vi "WAM_UserInput_Popup.vi"(0 "Enable":bool=TRUE, 5 "error in (no error)":errorcluster, 11 "UseBcScanner(t)":bool=TRUE) -> (8 "EmpName":string caption="Revision", 10 "UserString":string="062218\r\n", 12 "operator infor header":string, 14 "UserInput_Popup_refOut":refnum<vi>, 17 "UserBCPopup_ref_out":refnum<vi>, 18 "OK":bool, 19 "error out":errorcluster)   [LabVIEW 2018]
doc: "Displays a standard dialog box that prompts users to enter information, such as a user name and password.\n--------------------\n\nThis Express VI is configured as follows:\n\nMessage to Display to the User:"
panel:
  out "index of element":i32=-1
  in  "EmpLocation":string(combo) caption="LotID"
  in  "EmpName":string caption="Revision"
  in  "EmpID#":string caption="PN"
  out "String":string
  in  "Cancel":bool=TRUE
  in  "OK2":bool
  in  "OK1":bool=TRUE
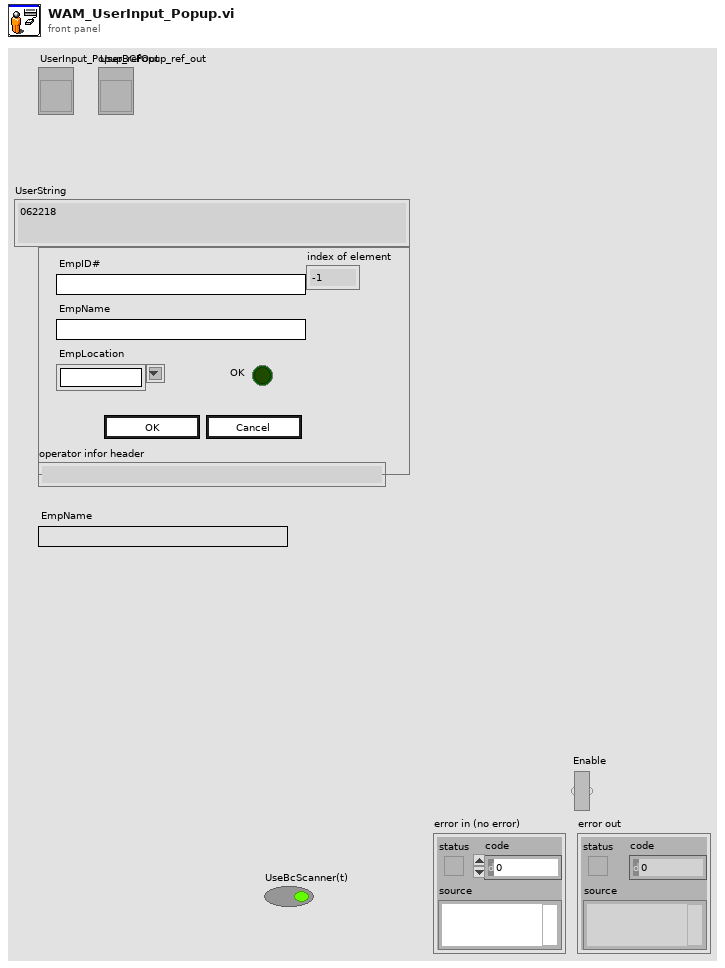
[diagram p1: front panel]
types:
  T1 = cluster{"Input Name":string, "Input Data Type":i32}[]
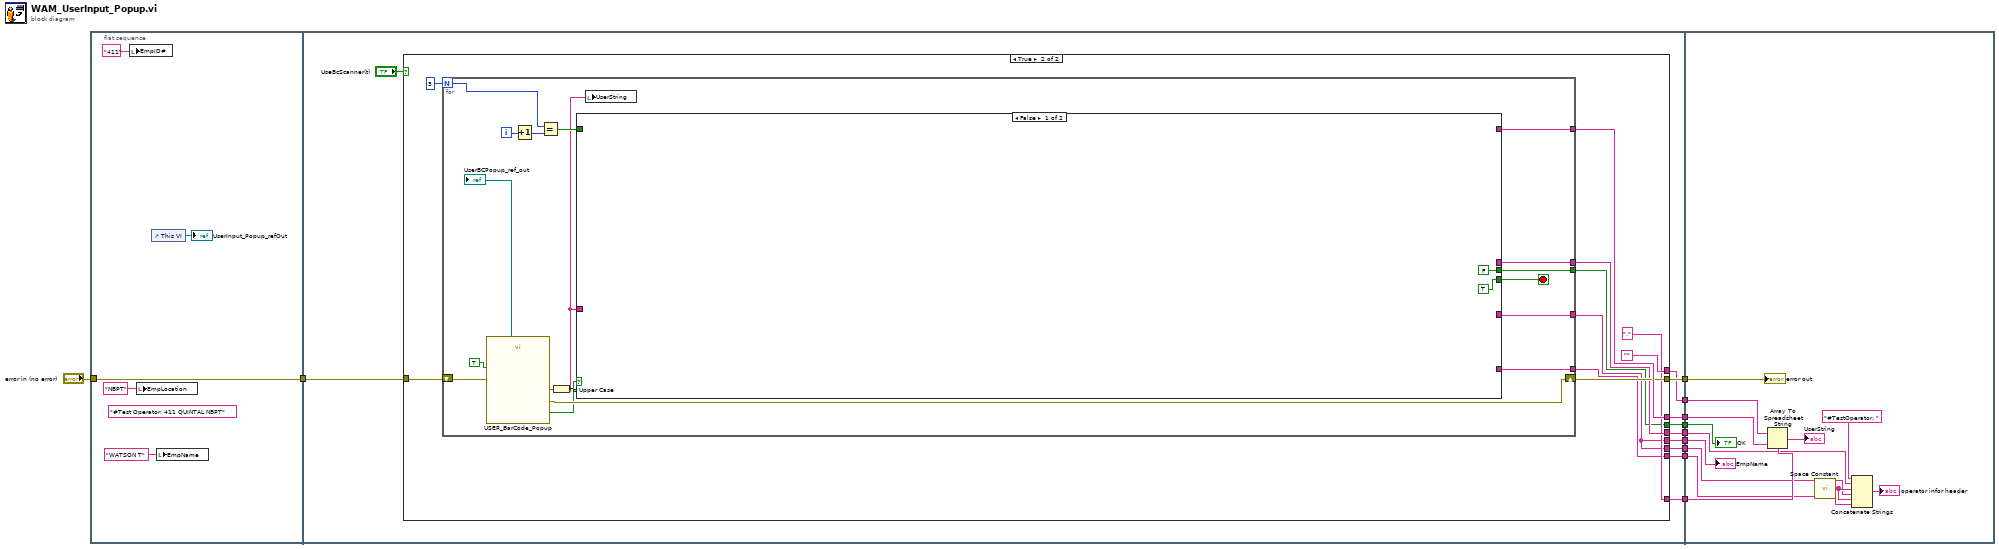
[diagram p0: block diagram]
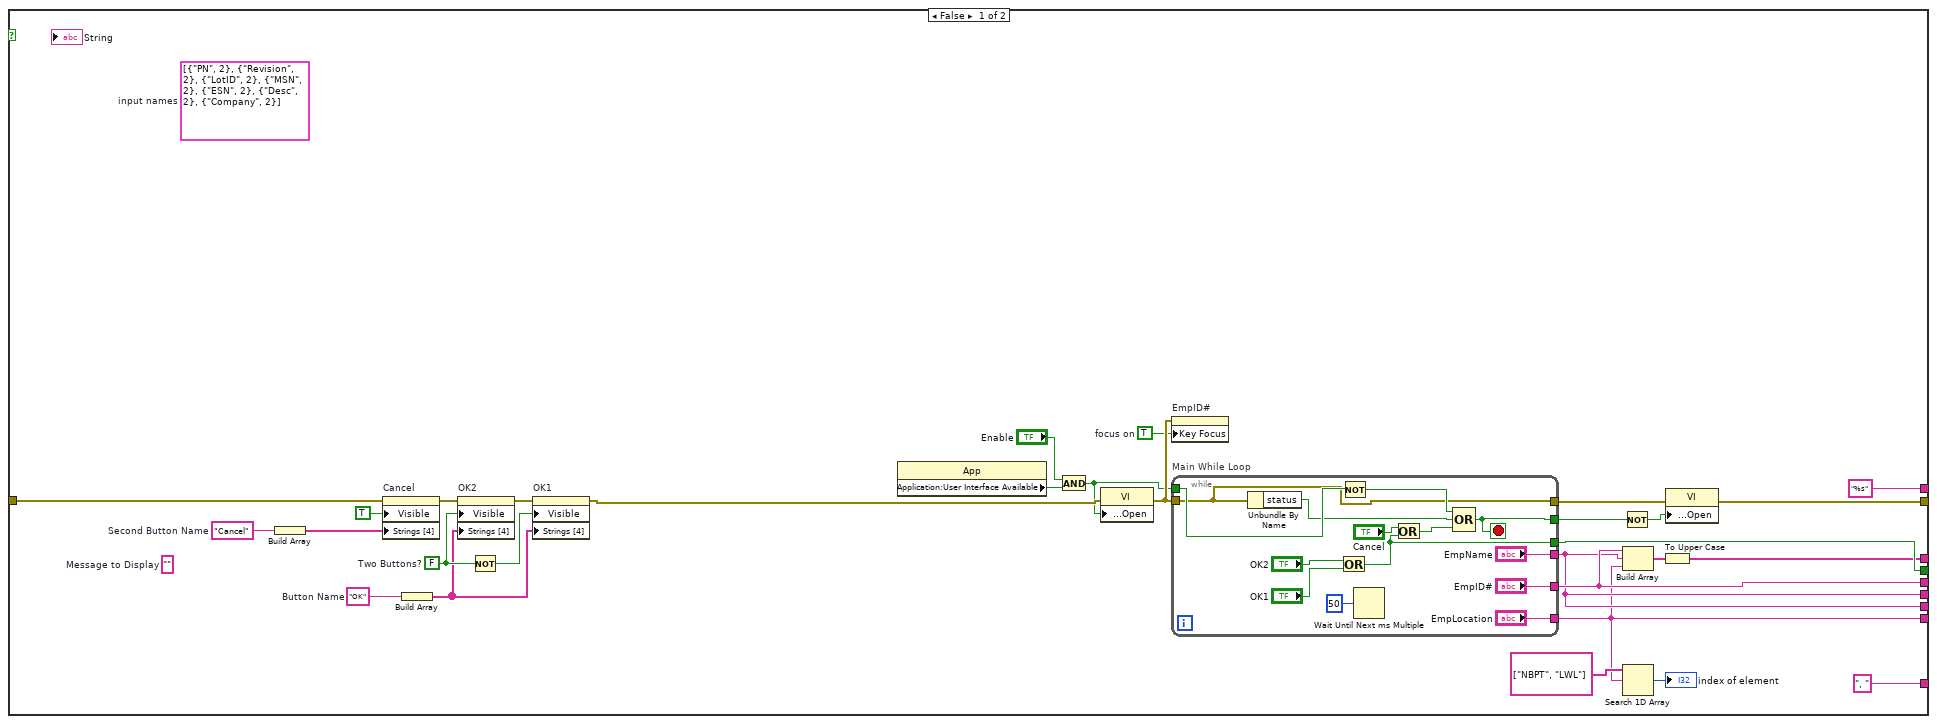
[diagram p2: hidden frame]
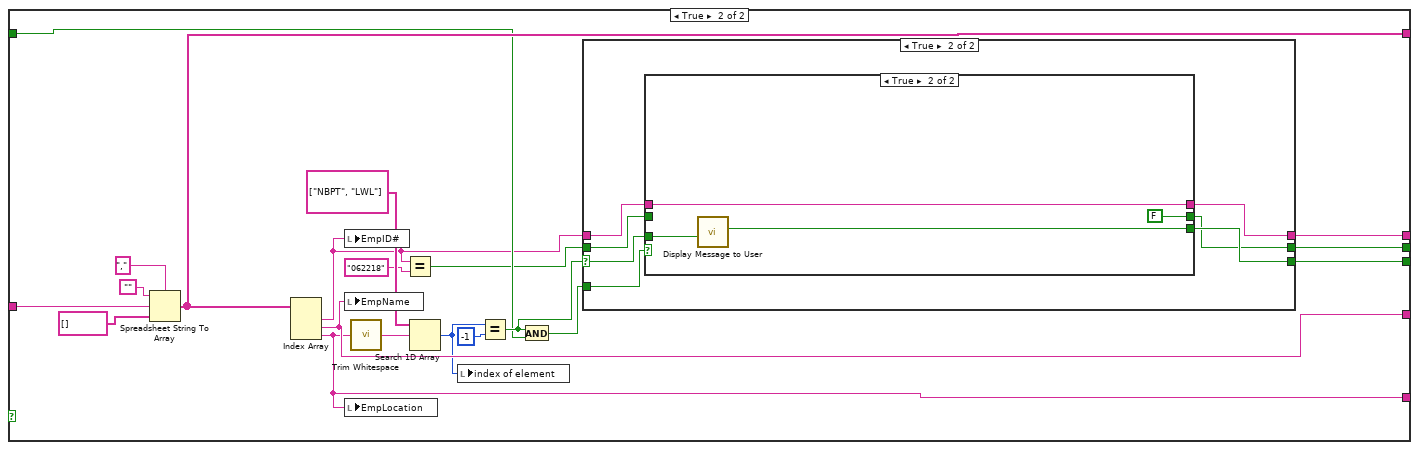
[diagram p3: hidden frame]
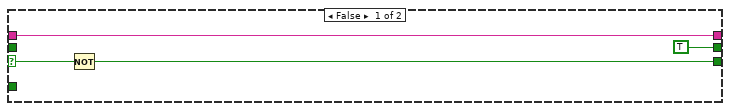
[diagram p4: hidden frame]
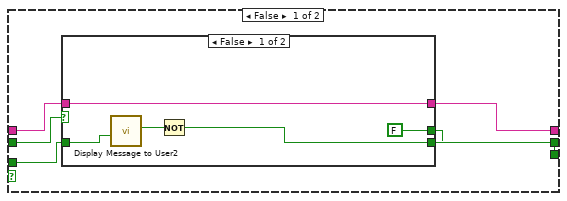
[diagram p5: hidden frame]
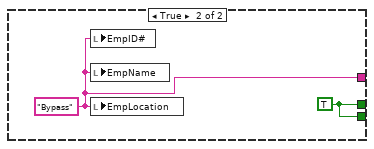
[diagram p6: hidden frame]
diagram:
  n1 = flat-sequence {
    tunnel: "error in (no error)" -> [w16]
    tunnel: [w16] -> w10
    tunnel: w10 -> [w27]
    tunnel: [w26] -> w9
    tunnel: [w25] -> w8
    tunnel: [w24] -> w7
    tunnel: [w23] -> w6
    tunnel: [w22] -> w5
    tunnel: [w20] -> w4
    tunnel: [w19] -> w3
    tunnel: [w18] -> w2
    tunnel: [w17] -> w1
    tunnel: w9 -> [w160]
    tunnel: w8 -> [w158]
    tunnel: w7 -> [w154]
    tunnel: w6 -> [w152]
    tunnel: w5 -> [w151]
    tunnel: w4 -> [w157]
    tunnel: w3 -> [w159]
    tunnel: w2 -> [w156]
    tunnel: w1 -> [w161]
    frame #0 {
      (unwired) "#Test Operator: 411 QUINTAL NBPT" ("OperatorInfo")
      n2 = local write "EmpID#"("411" ("PN")) -> ()
      n3 = local write "EmpLocation"("NBPT" ("LotID")) -> ()
      n4 = control-ref of="This VI"() -> (→"UserInput_Popup_refOut":refnum<vi>)
      n5 = local write "EmpName"("WATSON T" ("Revision")) -> ()
    }
    frame #1 {
      n6 = case shown="True" "UseBcScanner(t)" {
        tunnel: w27 -> [w45 w80]
        tunnel: [w43 w79] -> w26
        tunnel: [w28 w81] -> w25
        tunnel: [w36 w78] -> w24
        tunnel: [w33 w75] -> w23
        tunnel: [w31 w74] -> w22
        tunnel: ["%s" ("format string") "" ("format string")] -> w20
        tunnel: [", " ("delimiter (Tab)") "," ("delimiter (Tab)")] -> w19
        tunnel: [w33 w75] -> w18
        tunnel: [w29 w72] -> w17
        frame False {
          w39 = TRUE  # focus on
          (unwired) T1 [{"Input Name"="PN", "Input Data Type"=2}, {"Input Name"="Revision", "Input Data Type"=2}, {"Input Name"="LotID", "Input Data Type"=2}, {"Input Name"="MSN", "Input Data Type"=2}, {"Input Name"="ESN", "Input Data Type"=2}, {"Input Name"="Desc", "Input Data Type"=2}, {"Input Name"="Company", "Input Data Type"=2}]  # input names
          w50 = "Cancel"  # Second Button Name
          w48 = "OK"  # Button Name
          (unwired) ""  # Message to Display
          w57 = FALSE  # Two Buttons?
          n7 = Build Array(w50) -> (w51:string[])
          n8 = property on="Cancel" class="Bool"(error in=w45, "Visible"=TRUE, "Strings [4]"=w51) -> (error out=w55:errorcluster)  [unwired: 1 in, 1 out]
          n9 = Build Array(w48) -> (w49:string[])
          n10 = property on="OK2" class="Bool"(error in=w55, "Visible"=w57, "Strings [4]"=w49) -> (error out=w54:errorcluster)  [unwired: 1 in, 1 out]
          n11 = Not(x=w57) -> (.not. x?=w56:bool)
          n12 = property on="OK1" class="Bool"(error in=w54, "Visible"=w56, "Strings [4]"=w49) -> (error out=w47:errorcluster)  [unwired: 1 in, 1 out]
          n13 = property class="App"() -> ("Application:User Interface Available"=w40:bool)  [unwired: 2 in, 2 out]
          n14 = And(x="Enable", y=w40) -> (x .and. y?=w41:bool)
          n15 = property class="VI"(error in=w47, "Front Panel Window:Open"=w41) -> (error out=w46:errorcluster)  [unwired: 1 in, 1 out]
          n16 = property on="EmpID#" class="Str"(error in=w46, "Key Focus"=w39) -> ()  [unwired: 1 in, 2 out]
          n17 = while "Main While Loop" {
            tunnel: [w68] -> w29
            tunnel: w41 -> [w66]
            tunnel: [w64] -> w52
            tunnel: w46 -> [w63]
            tunnel: [w63] -> w44
            tunnel: ["EmpID#"] -> w36
            tunnel: ["EmpName"] -> w33
            tunnel: ["EmpLocation"] -> w31
            stop <- w64 stop-if-true
            n18 = Unbundle By Name(w63) -> ("status"=w61:bool)
            n19 = Or(x="OK2", y="OK1") -> (x .or. y?=w68:bool)
            n20 = Not(x=w66) -> (.not. x?=w65:bool)
            n21 = Wait Until Next ms Multiple(millisecond multiple=u32 50) -> ()  [unwired: 1 out]
            n22 = Or(x="Cancel", y=w68) -> (x .or. y?=w62:bool)
            n23 = Compound Arithmetic op=OR(w65, w61, w62) -> (w64:bool)
          }
          n24 = Not(x=w52) -> (.not. x?=w53:bool)
          n25 = Build Array(w36, w33, w31) -> (w38:string[])
          n26 = Search 1D Array(1D array=string[] ["NBPT", "LWL"], element=w31) -> (index of element=→"index of element":i32)  [unwired: 1 in]
          n27 = To Upper Case(1:w38) -> (0:w28:string[])
          n28 = property class="VI"(error in=w44, "Front Panel Window:Open"=w53) -> (error out=w43:errorcluster)  [unwired: 1 in, 1 out]
        }
        frame True {
          n29 = for {
            N: 3 -> [w91]
            tunnel: [w97] -> w81
            tunnel: [w88] -> w78
            tunnel: [w94] -> w75
            tunnel: [w93] -> w74
            shift-right: [w95] -> w79
            shift-left: w80 -> [w96]
            tunnel: [w85] -> w72
            i -> [w90]
            stop <- w87 stop-if-true
            n30 = call "USER_BarCode_Popup.vi"("Enable"=TRUE, "error in (no error)"=w96) -> ("UserBCPopup_ref_out"=→"UserBCPopup_ref_out":refnum<vi>, "Bar Code"=w84:string, "OK"=w86:bool, "error out"=w95:errorcluster)  [unwired: 14 in]
            n31 = Increment(x=w90) -> (x+1=w89:i32)
            n32 = Equal?(x=w91, y=w89) -> (x = y?=w92:bool)
            n33 = To Upper Case(1:w84) -> (0:w82:string)
            n34 = case shown="False" w86 {
              tunnel: w82 -> [_ w119]
              tunnel: [_ w117] -> w97
              tunnel: [_ w115] -> w94
              tunnel: [_ w113] -> w93
              tunnel: w92 -> [_ w108]
              tunnel: [_ w104] -> w88
              tunnel: [TRUE ("OK") w102] -> w87
              tunnel: [FALSE ("OK") w101] -> w85
              frame False {
              }
              frame True {
                n35 = Spreadsheet String To Array(delimiter (Tab)=",", format string="", spreadsheet string=w119, array type (2D Dbl)=string[] []) -> (array=w117:string[])
                n36 = Index Array(array=w117) -> (element #1=w103:string, element #2=w115:string, element #3=w113:string)  [unwired: 3 in]
                n37 = local write "EmpID#"(w103) -> ()
                n38 = local write "EmpName"(w115) -> ()
                n39 = local write "EmpLocation"(w113) -> ()
                n40 = call <vilib>:"Trim Whitespace.vi"("string"=w113) -> ("trimmed string"=w110:string)  [unwired: 1 in]
                n41 = Equal?(x=w103, y="062218") -> (x = y?=w105:bool)
                n42 = Search 1D Array(1D array=string[] ["NBPT", "LWL"], element=w110) -> (index of element=w112:i32)  [unwired: 1 in]
                n43 = local write "index of element"(w112) -> ()
                n44 = Equal?(x=w112, y=-1) -> (x = y?=w109:bool)
                n45 = And(x=w109, y=w108) -> (x .and. y?=w107:bool)
                n46 = case shown="True" w109 {
                  selector: w109 -> [w124 w131]
                  tunnel: [w123 w130] -> w102
                  tunnel: w107 -> [_ w129]
                  tunnel: w105 -> [_ w128]
                  tunnel: [w122 w127] -> w104
                  tunnel: w103 -> [w122 w126]
                  tunnel: [TRUE w125] -> w101
                  frame False {
                    n47 = Not(x=w124) -> (.not. x?=w123:bool)
                  }
                  frame True {
                    n48 = case shown="True" w129 {
                      tunnel: w131 -> [w137 w148]
                      tunnel: [w136 w147] -> w130
                      tunnel: w128 -> [w135 _]
                      tunnel: [w134 w146] -> w127
                      tunnel: w126 -> [w133 w146]
                      tunnel: [w132 FALSE] -> w125
                      frame False {
                        n49 = case shown="False" w135 {
                          tunnel: w137 -> [w142 _]
                          tunnel: [w140 w143] -> w136
                          tunnel: [w139 w144] -> w134
                          tunnel: w133 -> [w139 _]
                          tunnel: [FALSE w143] -> w132
                          frame False {
                            n50 = call "Display Message to User2"("Enable"=w142) -> ("OK"=w141:bool)  [unwired: 9 in, 1 out]
                            n51 = Not(x=w141) -> (.not. x?=w140:bool)
                          }
                          frame True {
                            w144 = "Bypass" ("EmpName")
                            w143 = TRUE
                            n52 = local write "EmpID#"(w144) -> ()
                            n53 = local write "EmpName"(w144) -> ()
                            n54 = local write "EmpLocation"(w144) -> ()
                          }
                        }
                      }
                      frame True {
                        n55 = call "Display Message to User"("Enable"=w148) -> ("OK"=w147:bool)  [unwired: 9 in, 1 out]
                      }
                    }
                  }
                }
              }
            }
            n56 = local write "UserString"(w82) -> ()
          }
        }
      }
    }
    frame #2 {
      n57 = Array To Spreadsheet String(delimiter (Tab)=w159, array=w158, 3:w157) -> (spreadsheet string=→"UserString":string)
      n58 = call <vilib>:"Space Constant.vi"() -> ("String"=w153:string)
      n59 = Concatenate Strings("#TestOperator: " ("string"), w154, w153, w152, w153, w151) -> (→"operator infor header":string)
      "OK" <- w161
      "error out" <- w160
      "EmpName" <- w156
    }
  }
